vi "Change Pump Setpoint.vi"(6 "timeout (1000 ms)":i32=1000, 8 "error in (no error)":errorcluster, 10 "Pump Setpoint":dbl, 11 "PolyA in":refnum<class "System.lvclass">) -> (0 "error out":errorcluster, 2 "Setpoint":dbl, 3 "PolyA out":refnum<class "System.lvclass">, 4 "timed out?":bool)   [LabVIEW 2014, in "System.lvclass"]
doc: "For polynomial coefficients = [a, b, c]\nP(x) = a + b*(x^1) + c*(x^2)"
uses:
  System.lvclass
  Query Payload -- cluster.ctl
  System.lvclass/System.ctl
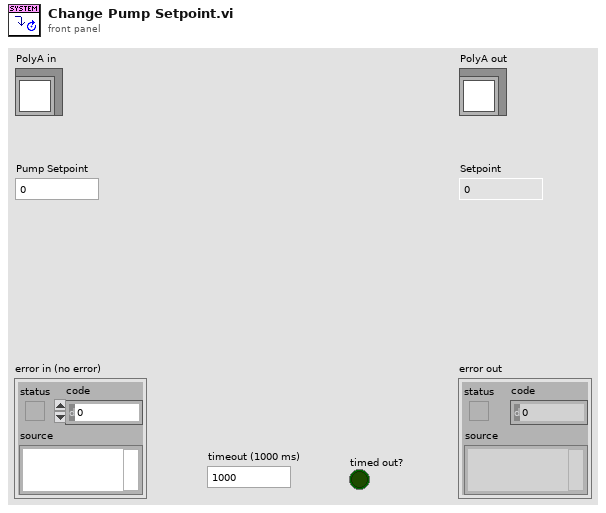
[diagram p1: front panel]
types:
  T1 = typedef "System.lvclass/Query Payload -- cluster.ctl" = cluster{"setpoint":dbl, "notifier":refnum<notifier>}
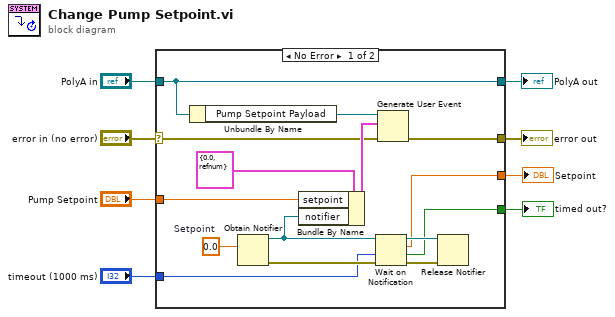
[diagram p0: block diagram]
diagram:
  n1 = case shown="No Error" "error in (no error)" {
    selector: "error in (no error)" -> [w11 w25]
    tunnel: [w10 w25] -> w7
    tunnel: [w17 w24] -> w5
    tunnel: "PolyA in" -> [w17 w24]
    tunnel: "timeout (1000 ms)" -> [w21 _]
    tunnel: [w18 _] -> w3
    tunnel: "Pump Setpoint" -> [w14 _]
    tunnel: [w9 _] -> w1
    frame No Error {
      w23 = 0.0  # Setpoint
      n2 = Unbundle By Name(w17) -> ("Pump Setpoint Payload"=w16:refnum<user-event>)
      n3 = Obtain Notifier(notification data type=w23) -> (notifier out=w13:refnum<notifier>, error out=w22:errorcluster)  [unwired: 3 in, 1 out]
      n4 = Bundle By Name(cluster=T1 {"setpoint"=0.0, "notifier"=refnum} ("Query Payload"), "setpoint"=w14, "notifier"=w13) -> (w12:T1)
      n5 = Wait on Notification(notifier=w13, timeout in ms (-1)=w21, error in (no error)=w22) -> (notifier out=w20:refnum<notifier>, notification=w18:dbl, timed out?=w9:bool, error out=w19:errorcluster)  [unwired: 1 in]
      n6 = Generate User Event(user event=w16, event data cluster=w12, error in=w11) -> (error out=w10:errorcluster)  [unwired: 1 in, 1 out]
      n7 = Release Notifier(notifier=w20, error in (no error)=w19) -> ()  [unwired: 1 in, 3 out]
    }
    frame Error {
    }
  }
  "error out" <- w7
  "PolyA out" <- w5
  "Setpoint" <- w3
  "timed out?" <- w1
